vi "Add Timer.vi"(8 "error in (no error)":errorcluster, 10 "Timer Config":T1={"Name"="", "Period [s]"=0.0, "Enabled"=TRUE, "Metadata"=""}, 11 "Task Scheduler Actor in":refnum<class "Task Scheduler Actor.lvclass">) -> (0 "error out":errorcluster, 3 "Task Scheduler Actor out":refnum<class "Task Scheduler Actor.lvclass">)   [LabVIEW 2015, in "Task Scheduler Actor.lvclass"]
uses:
  Task Scheduler Actor.lvclass
  Timer Config.ctl
  Task Scheduler Actor.lvclass/Task Scheduler Actor.ctl
  Re-use Libraries/Timer/Timer.lvclass/Timer.ctl
  Re-use Libraries/Timer/Timer.lvclass
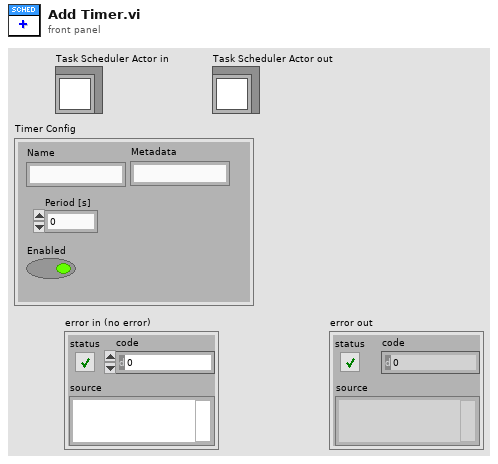
[diagram p1: front panel]
types:
  T1 = typedef "Task Scheduler Actor.lvclass/Timer Config.ctl" = cluster{"Name":string, "Period [s]":dbl, "Enabled":bool, "Metadata":string}
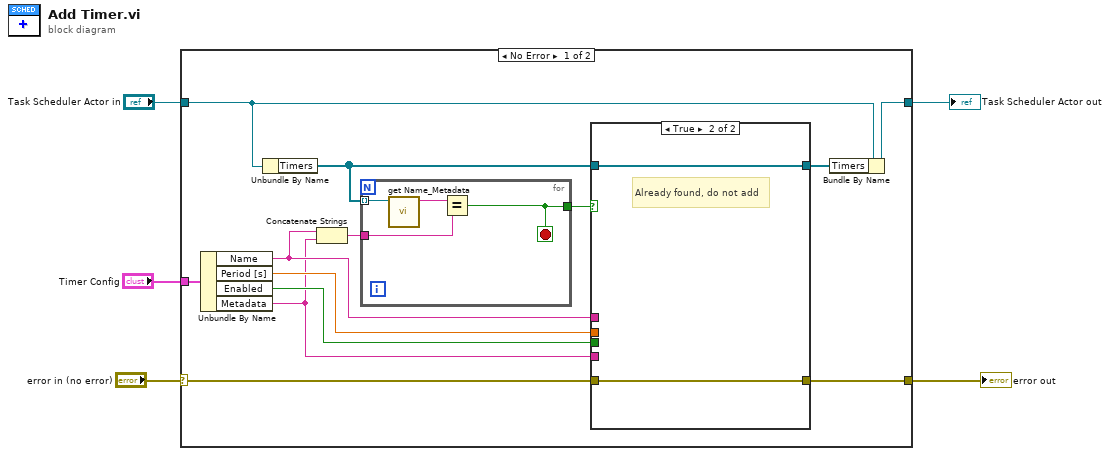
[diagram p0: block diagram]
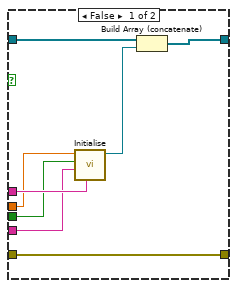
[diagram p2: hidden frame]
diagram:
  n1 = case shown="No Error" "error in (no error)" {
    selector: "error in (no error)" -> [w12 w34]
    tunnel: [w17 w33] -> w5
    tunnel: "Task Scheduler Actor in" -> [w16 w33]
    tunnel: "Timer Config" -> [w11 _]
    tunnel: [w13 w34] -> w2
    frame No Error {
      n2 = Unbundle By Name(w11) -> ("Name"=w8:string, "Period [s]"=w10:dbl, "Enabled"=w9:bool, "Metadata"=w7:string)
      n3 = Unbundle By Name(w16) -> ("Timers"=w15:refnum<class "Timer.lvclass">[])
      n4 = Concatenate Strings(w8, w7) -> (w6:string)
      n5 = for {
        tunnel: w15 -> [w31] mode=indexing
        tunnel: [w32] -> w14
        tunnel: w6 -> [w29]
        stop <- w32 stop-if-true
        n6 = call "get Name_Metadata .vi"("Timer in"=w31) -> ("Name"=w30:string)  [unwired: 10 in]
        n7 = Equal?(x=w30, y=w29) -> (x = y?=w32:bool)
      }
      n8 = case shown="True" w14 {
        tunnel: w8 -> [w26 _]
        tunnel: w15 -> [w25 w28]
        tunnel: [w23 w28] -> w18
        tunnel: [w22 w27] -> w13
        tunnel: w12 -> [w22 w27]
        tunnel: w10 -> [w21 _]
        tunnel: w9 -> [w20 _]
        tunnel: w7 -> [w19 _]
        frame False {
          n9 = call "Initialise.vi"("Name"=w26, "Metadata"=w19, "Enabled (T)"=w20, "Period [s]"=w21) -> ("Timer out"=w24:refnum<class "Timer.lvclass">)  [unwired: 7 in]
          n10 = Build Array (concatenate)(w25, w24) -> (w23:refnum<class "Timer.lvclass">[])
        }
        frame True {
          # "Already found, do not add"
        }
      }
      n11 = Bundle By Name(cluster=w16, "Timers"=w18) -> (w17:refnum<class "Task Scheduler Actor.lvclass">)
    }
    frame Error {
    }
  }
  "Task Scheduler Actor out" <- w5
  "error out" <- w2
